vi "Get SMO Name.vi"(8 "error in (no error)":errorcluster, 11 "RP100 in":refnum<class "RP100.lvclass">) -> (0 "error out":errorcluster, 2 "SMO Name":string, 3 "RP100 out":refnum<class "RP100.lvclass">)   [LabVIEW 2019, in "RP100.lvclass"]
uses:
  RP100.lvclass
  <userlib>/LevyLab/Instrument Framework/Instrument Types/Strain/Instrument.Strain.lvclass
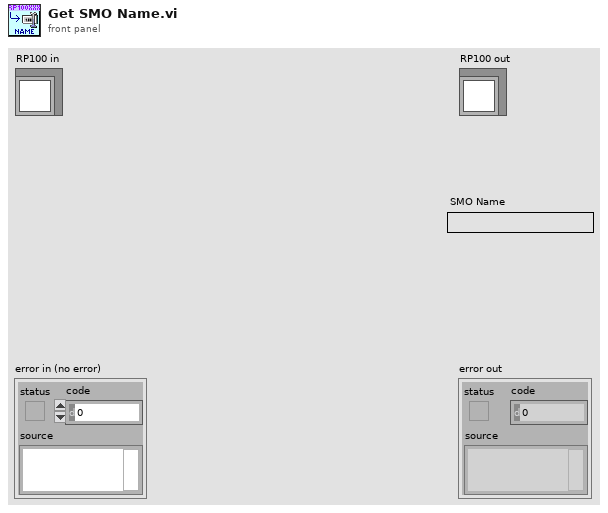
[diagram p1: front panel]
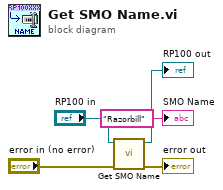
[diagram p0: block diagram]
diagram:
  n1 = call-parent "Get SMO Name.vi"("error in (no error)"="error in (no error)", "Instrument in"="RP100 in") -> ("error out"=→"error out":errorcluster, "Instrument out"=→"RP100 out":refnum<class "RP100.lvclass">)  [unwired: 7 in, 1 out]
  "SMO Name" <- "Razorbill" ("SMO Name")
